vi "poly_is_specific_control_NumericWithScale.vi"(2 "ctrl ref":refnum<vi>) -> (7 "is NumericWithScale?":bool)   [LabVIEW 2015]
uses:
  cores/core_controls_children_names.ctl
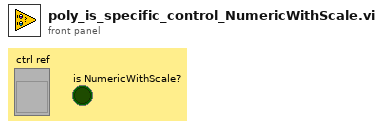
[diagram p1: front panel]
types:
  T1 = typedef "core_controls_children_names.ctl" = enum16{"AbsTime", "ActiveXContainer", "Array", "Boolean", "Cluster", "RadioButtonsControl", "ColorBox", "DigitalTable", "GraphChart", "IntensityChart", "IntensityGraph", "MixedSignalGraph", "WaveformChart", "WaveformGraph", "DigitalGraph", "XYGraph", "IOName", "DAQChannelName", "DAQmxName", "IVILogicalName", "VISAResourceName", "LabVIEWClassControl", "ListBox", "LVVariant", "MixedCheckbox", "MulticolumnListbox", "MultiSegmentPipe", "Numeric", "ColorRamp", "Digital", "NamedNumeric", "Enum", "Ring", "NumericWithScale", "Knob", "Slide", "PageSelector", "TabControl", "Path", "Picture", "Pixmap", "RefNum", "LVObjectRefNum", "VIRefNum", "TypedRefNum", "DataValRefNum", "SceneGraphDisplay", "Scrollbar", "String", "ComboBox", "SubPanel", "Table", "TreeControl", "WaveformData"}
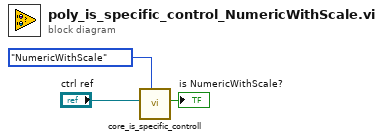
[diagram p0: block diagram]
diagram:
  n1 = call "core_is_specific_controll.vi"("specific class"=core_controls_children_names."NumericWithScale", "ctrl ref"="ctrl ref") -> ("is specific control?"=→"is NumericWithScale?":bool)  [unwired: 9 in]
